vi "ThorLabs Test.vi"() -> ()   [LabVIEW 2024]
uses:
  C:/Users/goods/OneDrive/Desktop/Work/program/MOVER/Thorlabs.MotionControl.TCube.DCServoCLI.dll
  Thorlabs.MotionControl.TCube.DCServoCLI.dll
  C:/Users/goods/OneDrive/Desktop/Work/program/MOVER/Thorlabs.MotionControl.Controls.dll
  Thorlabs.MotionControl.Controls.dll
panel:
  in  "TCubeDCServoControl":refnum<k24>(container)
  out "GetPositionCounter":dbl
  in  "stop":bool
  in  "SerialNumber":string
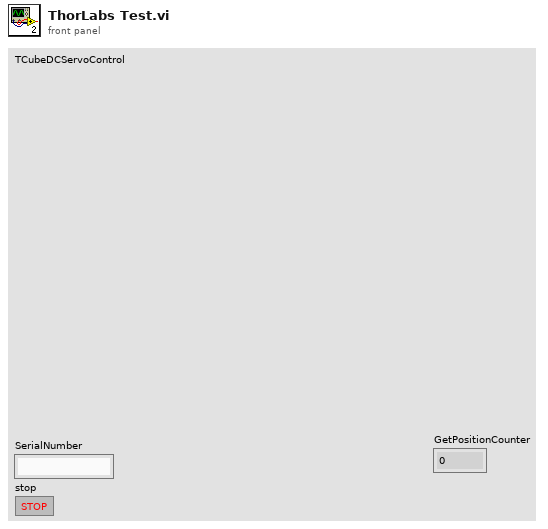
[diagram p1: front panel]
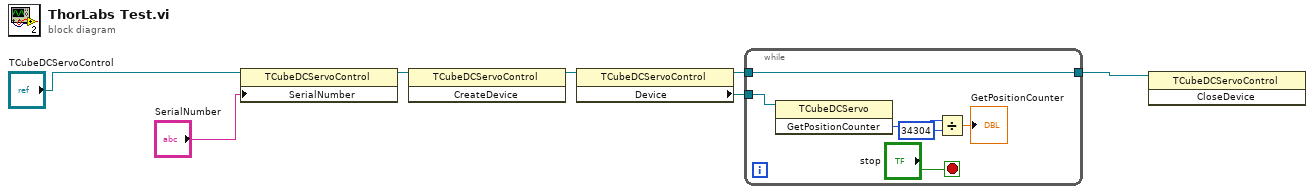
[diagram p0: block diagram]
diagram:
  n1 = property class="TCubeDCServoControl"(reference="TCubeDCServoControl", "SerialNumber"="SerialNumber") -> (reference out=w6:refnum<k24>)  [unwired: 1 in, 1 out]
  n2 = invoke class="TCubeDCServoControl" method="CreateDevice"(reference=w6) -> (reference out=w5:refnum<k24>)  [unwired: 2 in, 2 out]
  n3 = property class="TCubeDCServoControl"(reference=w5) -> (reference out=w2:refnum<k24>, "Device"=w3:refnum<k24>)  [unwired: 1 in, 1 out]
  n4 = while {
    tunnel: [w11] -> w4
    tunnel: w3 -> [w12]
    tunnel: w2 -> [w11]
    stop <- "stop" stop-if-true
    n5 = invoke class="TCubeDCServo" method="GetPositionCounter"(reference=w12) -> ("GetPositionCounter"=w10:i32)  [unwired: 2 in, 2 out]
    n6 = Divide(x=w10, y=34304) -> (x/y=→"GetPositionCounter":dbl)
  }
  n7 = invoke class="TCubeDCServoControl" method="CloseDevice"(reference=w4) -> ()  [unwired: 2 in, 3 out]
